vi "return to start sub.vi"(5 "Set speed":dbl, 6 "Return to start":bool, 7 "Current position in":dbl, 8 "Stepper 0 error in":errorcluster, 9 "Stepper 0 in":T1, 10 "Pin 2 error in":errorcluster, 11 "Pin 2 in":T1) -> (0 "Stepper 0 error out":errorcluster, 1 "Stepper 0 out":T1, 2 "Pin 2 error out":errorcluster, 3 "Pin 2 out":T1, 4 "Current position out":dbl)   [LabVIEW 2018]
uses:
  <vilib>/LabVIEW Interface for Arduino/Type Defs/Arduino Resource.ctl
  <vilib>/LabVIEW Interface for Arduino/Type Defs/Board Type.ctl
  <vilib>/LabVIEW Interface for Arduino/LabVIEW Interface for Arduino.lvlib
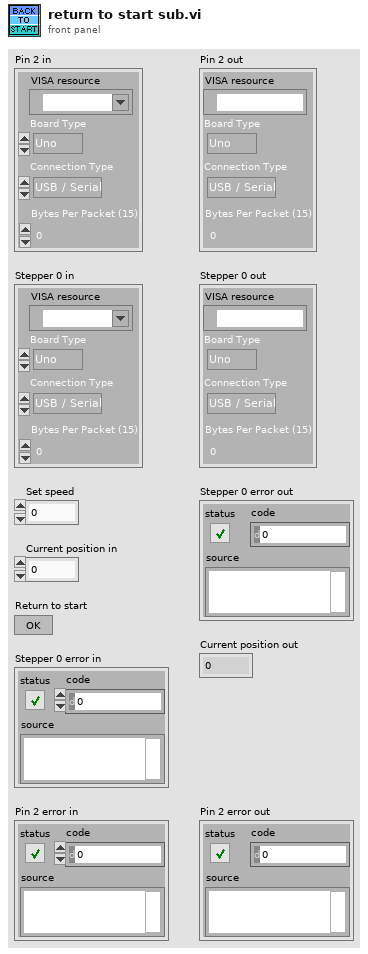
[diagram p1: front panel]
types:
  T1 = typedef "LabVIEW Interface for Arduino.lvlib/Arduino Resource.ctl" = cluster{"VISA resource":refnum<visa-resource-name>, "Board Type":T2, "Connection Type":enum8{"USB / Serial"}, "Bytes Per Packet (15)":u8}
  T2 = typedef "LabVIEW Interface for Arduino.lvlib/Board Type.ctl" = enum16{"Uno", "Dimuelanove w/Atmega 328", "Mega 2560"}
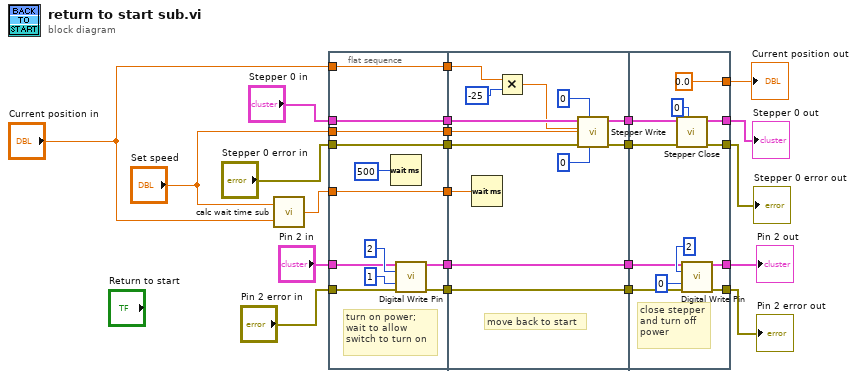
[diagram p0: block diagram]
diagram:
  n1 = call "calc wait time sub.vi"("mm to go"="Current position in", "set speed (steps/s)"="Set speed") -> ("wait time"=w12:dbl)
  n2 = flat-sequence {
    tunnel: "Stepper 0 error in" -> [w27]
    tunnel: "Set speed" -> [w35]
    tunnel: "Stepper 0 in" -> [w28]
    tunnel: [w35] -> w23
    tunnel: "Pin 2 in" -> [w32]
    tunnel: "Pin 2 error in" -> [w31]
    tunnel: [w30] -> w22
    tunnel: [w29] -> w21
    tunnel: [w28] -> w20
    tunnel: [w27] -> w19
    tunnel: [w25] -> w18
    tunnel: w12 -> [w25]
    tunnel: "Current position in" -> [w24]
    tunnel: [w24] -> w1
    tunnel: [w46] -> w17
    tunnel: [w45] -> w16
    tunnel: w23 -> [w39]
    tunnel: [w41] -> w15
    tunnel: w22 -> [w41]
    tunnel: [w40] -> w14
    tunnel: w21 -> [w40]
    tunnel: w20 -> [w43]
    tunnel: w19 -> [w42]
    tunnel: w18 -> [w37]
    tunnel: w1 -> [w36]
    tunnel: w17 -> [w54]
    tunnel: w16 -> [w53]
    tunnel: [w52] -> w4
    tunnel: [w59] -> w6
    tunnel: [w58] -> w13
    tunnel: w15 -> [w57]
    tunnel: w14 -> [w56]
    tunnel: [w51] -> w9
    tunnel: [0.0] -> w10
    frame #0 {
      # "turn on power;\nwait to allow \nswitch to turn on"
      n3 = Wait (ms)(milliseconds to wait=500) -> ()  [unwired: 1 out]
      n4 = call <vilib>:"Digital Write Pin.vi"("Arduino Resource"=w32, "Digital I/O Pin (0)"=2, "Value (0)"=1, "error in"=w31) -> ("Arduino Resource"=w30:T1, "error out"=w29:errorcluster)  [unwired: 10 in]
    }
    frame #1 {
      # "move back to start"
      n5 = Wait (ms)(milliseconds to wait=w37) -> ()  [unwired: 1 out]
      n6 = Multiply(x=w36, y=-25) -> (x*y=w38:dbl)
      n7 = call <vilib>:"Stepper Write.vi"("Set Acceleration (0 to disable)"=0, "Stepper #"=0, "error in"=w42, "Set Speed (Steps per Second)"=w39, "# of Steps to Move"=w38, "Arduino Resource"=w43) -> ("error out"=w45:errorcluster, "Arduino Resource Out"=w46:T1)  [unwired: 4 in]
    }
    frame #2 {
      # "close stepper\nand turn off\npower"
      n8 = call <vilib>:"Stepper Close.vi"("Stepper #"=0, "error in"=w53, "Arduino Resource"=w54) -> ("error out"=w52:errorcluster, "Arduino Resource Out"=w51:T1)  [unwired: 7 in]
      n9 = call <vilib>:"Digital Write Pin.vi"("Arduino Resource"=w57, "Digital I/O Pin (0)"=2, "Value (0)"=0, "error in"=w56) -> ("Arduino Resource"=w59:T1, "error out"=w58:errorcluster)  [unwired: 10 in]
    }
  }
  "Pin 2 error out" <- w13
  "Current position out" <- w10
  "Stepper 0 out" <- w9
  "Pin 2 out" <- w6
  "Stepper 0 error out" <- w4
